vi "Receive Results Object.vi"(8 "error in (no error)":errorcluster, 10 "Results.lvclass":refnum<class "Results.lvclass">, 11 "Measurement Setup in":refnum<class "Measurement Setup.lvclass">) -> (0 "error out":errorcluster, 3 "Measurement Setup out":refnum<class "Measurement Setup.lvclass">)   [LabVIEW 2017, in "Measurement Setup Controller.lvlib" / "Measurement Setup.lvclass"]
uses:
  Measurement Setup.lvclass
  C:/Program Files (x86)/National Instruments/LabVIEW 2017/user.lib/Common Components/Controller/Controller.lvclass
  <userlib>/Common Components/Results/Results.lvclass
  <userlib>/Common Components/Controller/Controller.lvclass
  <userlib>/Common Components/User Interface/Messages/Display Results/Display Results.lvclass
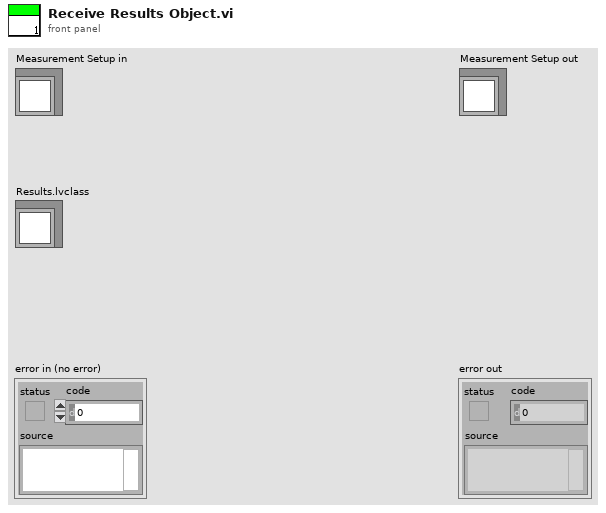
[diagram p1: front panel]
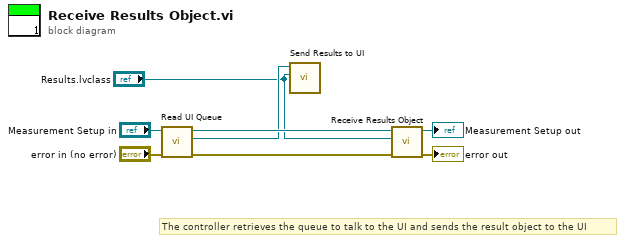
[diagram p0: block diagram]
diagram:
  # "The controller retrieves the queue to talk to the UI and sends the result object to the UI"
  n1 = call <userlib>:"Read UI Queue.vi"("error in (no error)"="error in (no error)", "UI Controller in"="Measurement Setup in") -> ("error out"=w1:errorcluster, "UI Queue"=w4:refnum<class "Message Enqueuer.lvclass">, "UI Controller out"=w5:refnum<class "Measurement Setup.lvclass">)  [unwired: 7 in]
  n2 = call <userlib>:"Send Results to UI.vi"("Results.lvclass"="Results.lvclass", "UI Queue"=w4) -> ()  [unwired: 8 in, 2 out]
  n3 = call-parent "Receive Results Object.vi"("error in (no error)"=w1, "Results.lvclass"="Results.lvclass", "Controller in"=w5) -> ("error out"=→"error out":errorcluster, "Controller out"=→"Measurement Setup out":refnum<class "Measurement Setup.lvclass">)  [unwired: 7 in]
